vi "Drag Start Row Visualization.vi"(7 "DragStart? (F)":bool, 8 "error in (no error)":errorcluster, 10 "DragStart Indices":i32[](array[numeric]), 11 "BetterBoxHandle in":refnum<class "BetterBoxHandle.lvclass">) -> (0 "error out":errorcluster, 3 "BetterBoxHandle out":refnum<class "BetterBoxHandle.lvclass">)   [LabVIEW 2020, in "BetterDragAndDrop.lvlib" / "BetterBoxHandle.lvclass"]
uses:
  BetterBoxHandle.lvclass
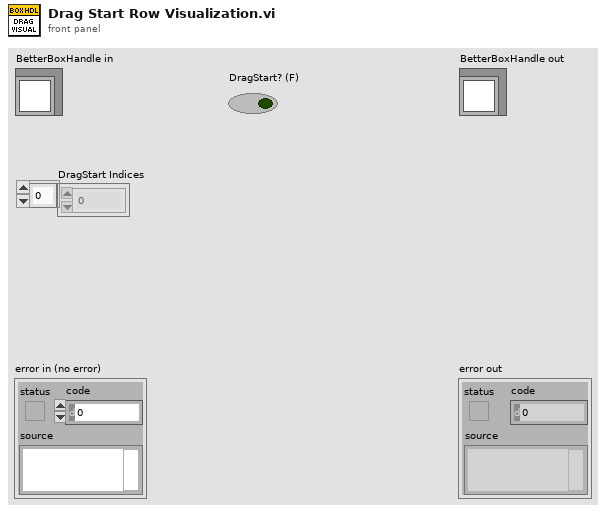
[diagram p1: front panel]
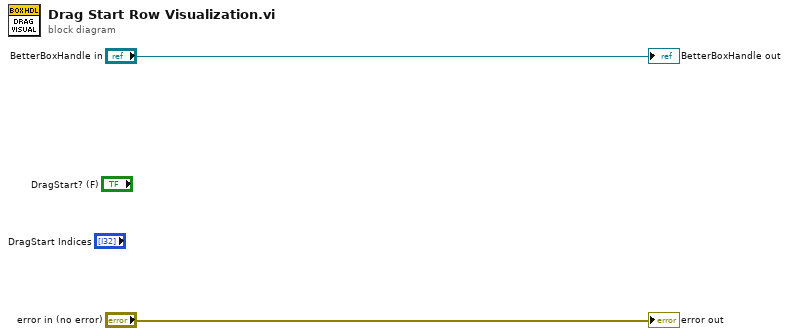
[diagram p0: block diagram]
diagram:
  "error out" <- "error in (no error)"
  "BetterBoxHandle out" <- "BetterBoxHandle in"
